vi "Timer data class VI - add times.vi"(0 "Timer in":refnum<class "Timer.lvclass">, 5 "Milliseconds":u32, 7 "Time 1":u32, 9 "Time 2":u32, 11 "error in (no error)":errorcluster) -> (4 "Timer out":refnum<class "Timer.lvclass">, 15 "error out":errorcluster)   [LabVIEW 2010, in "Timer.lvclass"]
uses:
  Timer.lvclass
  Timer.lvclass/Timer.ctl
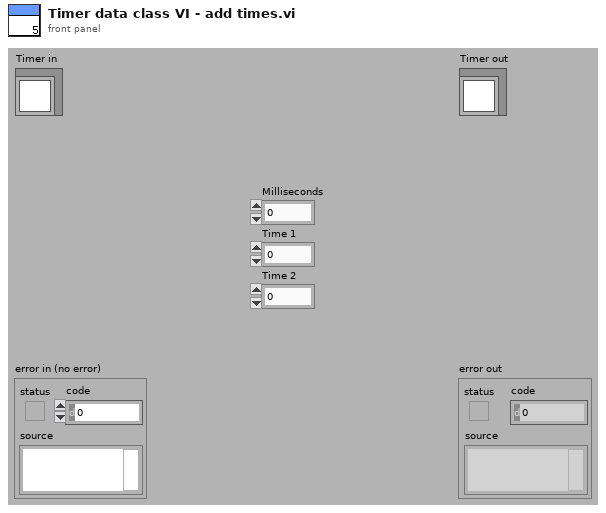
[diagram p1: front panel]
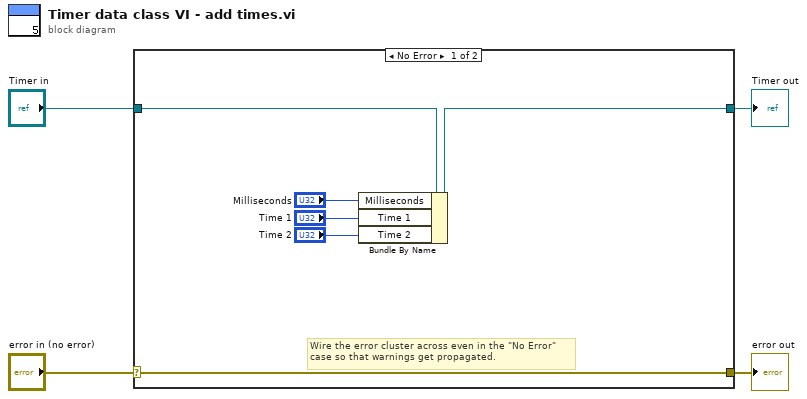
[diagram p0: block diagram]
diagram:
  n1 = case shown="No Error" "error in (no error)" {
    selector: "error in (no error)" -> [w9 w12]
    tunnel: [w9 w12] -> w3
    tunnel: [w8 w11] -> w1
    tunnel: "Timer in" -> [w10 w11]
    frame No Error {
      # "Wire the error cluster across even in the \"No Error\"\ncase so that warnings get propagated."
      n2 = Bundle By Name(cluster=w10, "Milliseconds"="Milliseconds", "Time 1"="Time 1", "Time 2"="Time 2") -> (w8:refnum<class "Timer.lvclass">)
    }
    frame Error {
    }
  }
  "error out" <- w3
  "Timer out" <- w1
